vi "XSens Verify Checksum (SubVI).vi"(11 "MTData2 Msg":string) -> (3 "CS Good?":bool)   [LabVIEW 2019]
doc: "Calculates the checksum of an Xsens MTData2 message. Message passed to this subvi must not include pre-ampnle byte (FA), but must include BID, MID, and DataLEN bytes. \n\nSums all bytes include the checksum byte, but not the preamble byte (per Xsens implementation). If LSB is zero, then message passes the checksum test and is presumed valid.\n\n2020 NREL"
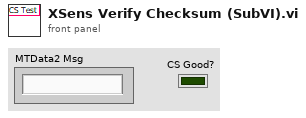
[diagram p1: front panel]
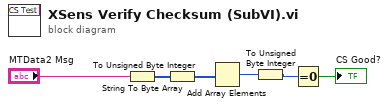
[diagram p0: block diagram]
diagram:
  n1 = String To Byte Array(string="MTData2 Msg") -> (unsigned byte array=w3:u8[])
  n2 = To Unsigned Byte Integer(number=w3) -> (unsigned 8bit integer=w4:u8[])
  n3 = Add Array Elements(numeric array=w4) -> (sum=w1:u8)
  n4 = To Unsigned Byte Integer(number=w1) -> (unsigned 8bit integer=w5:u8)
  n5 = Equal To 0?(x=w5) -> (x = 0?=→"CS Good?":bool)
